vi "XY Graph Load Single Column Plot from ASCII.vi"(8 "error in (no error)":errorcluster, 9 "Delimiter (TAB)":string="\t", 11 "String Array":string[](array[string])) -> (0 "error out":errorcluster, 1 "Single Column?":bool, 2 "Plot Array":cluster{"Array":dbl[], "Array":dbl[]}[](array[cluster]), 3 "String Array dup":string[](array[string]))   [LabVIEW 2019, in "XY Graph Add-Ons.lvlib"]
uses:
  XY Graph Add-Ons.lvlib
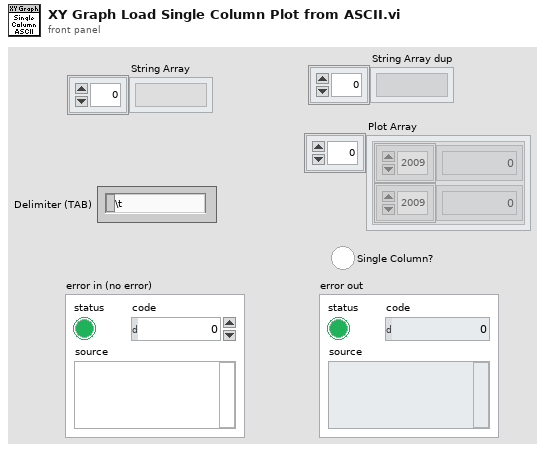
[diagram p1: front panel]
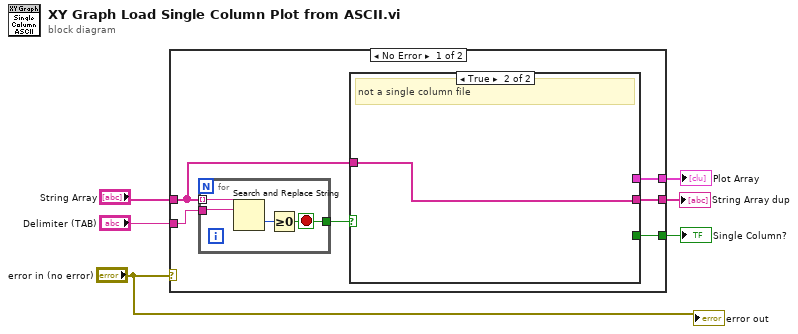
[diagram p0: block diagram]
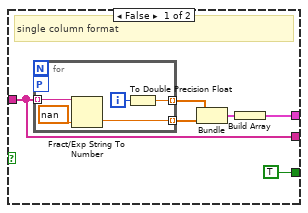
[diagram p2: hidden frame]
diagram:
  n1 = case shown="No Error" "error in (no error)" {
    tunnel: "Delimiter (TAB)" -> [w12 _]
    tunnel: [w11 _] -> w5
    tunnel: [w10 _] -> w4
    tunnel: "String Array" -> [w9 w29]
    tunnel: [w8 w29] -> w1
    frame No Error {
      n2 = for {
        tunnel: w12 -> [w16]
        tunnel: w9 -> [w15] mode=indexing
        tunnel: [w13] -> w7
        stop <- w13 stop-if-true
        n3 = Search and Replace String(input string=w15, search string=w16) -> (offset past replacement=w14:i32)  [unwired: 6 in, 3 out]
        n4 = Greater Or Equal To 0?(x=w14) -> (x >= 0?=w13:bool)
      }
      n5 = case shown="True" w7 {
        tunnel: w9 -> [w17 w28]
        tunnel: [w19 _] -> w11
        tunnel: [TRUE ("Single Column?") _] -> w10
        tunnel: [w17 w28] -> w8
        frame False {
          # "single column format"
          n6 = for {
            tunnel: w17 -> [w27] mode=indexing
            workers-P: _ -> [_]
            tunnel: [w25] -> w20 mode=indexing
            tunnel: [w23] -> w21 mode=indexing
            i -> [w24]
            n7 = Fract/Exp String To Number(string=w27, default (0 dbl)=nan ("default (0 DBL)")) -> (number=w25:dbl)  [unwired: 2 in, 1 out]
            n8 = To Double Precision Float(number=w24) -> (double precision float=w23:dbl)
          }
          n9 = Bundle(w21, w20) -> (w22:cluster{dbl[], dbl[]})  [unwired: 1 in]
          n10 = Build Array(w22) -> (w19:cluster{dbl[], dbl[]}[])
        }
        frame True {
          # "not a single column file"
        }
      }
    }
    frame Error {
    }
  }
  "Plot Array" <- w5
  "Single Column?" <- w4
  "String Array dup" <- w1
  "error out" <- "error in (no error)"
